vi "Save CITI File.vi"(8 "error in (no error)":errorcluster, 11 "CITI reference in":refnum<k24>) -> (0 "error out":errorcluster, 3 "CITI reference out":refnum<k24>)   [LabVIEW 2023, in "NI_HFNetworkAnalysis.lvlib"]
doc: "Save all CITI packages in memory to the referenced CITI file.\n\n<b>Notes</b>\n- If the referenced CITI file already exists, it is overwritten with the CITI packages in memory.\n- Use <b>Close CITI File.vi</b> to close reference to the CITI file."
uses:
  NI_HFNetworkAnalysis.lvlib
  C:/srd-semi-rfcal-software/AuxTools/STSRFFixtureCharactUtility/Source/Code Modules/Fixture/Dependencies/HFNetworkAnalysis/Support Files/NACE.Utils.Data.dll
  Support Files/NACE.Utils.Data.dll
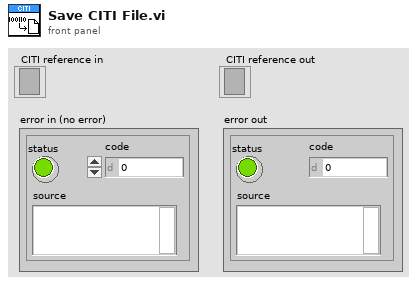
[diagram p1: front panel]
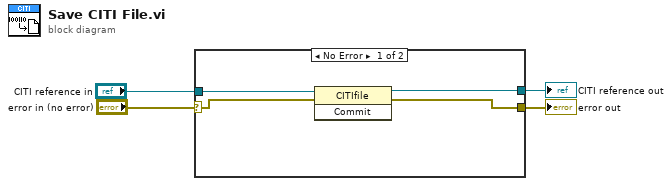
[diagram p0: block diagram]
diagram:
  n1 = case shown="No Error" "error in (no error)" {
    selector: "error in (no error)" -> [w7 w10]
    tunnel: "CITI reference in" -> [w8 w9]
    tunnel: [w6 w10] -> w2
    tunnel: [w5 w9] -> w1
    frame No Error {
      n2 = invoke class="CITIfile" method="Commit"(reference=w8, error in=w7) -> (reference out=w5:refnum<k24>, error out=w6:errorcluster)  [unwired: 1 in, 1 out]
    }
    frame Error {
    }
  }
  "error out" <- w2
  "CITI reference out" <- w1
